vi "F Dwf Analog Impedance Reference Get.vi"(8 "error in (no error)":errorcluster, 10 "pohms":dbl, 11 "hdwf":i32) -> (0 "error out":errorcluster, 2 "pohms out":dbl, 3 "function return":i32)   [LabVIEW 2019, in "Olasdwf.lvlib"]
doc: "DWFAPI int FDwfAnalogImpedanceReferenceGet(HDWF hdwf, double *pohms);"
uses:
  Olasdwf.lvlib
  Windows/System32/dwf.dll
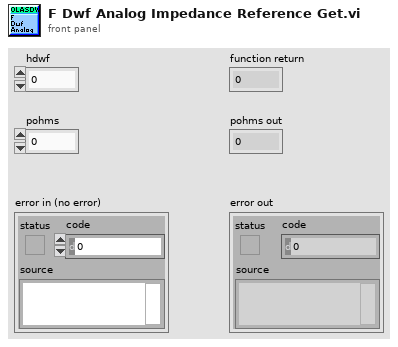
[diagram p1: front panel]
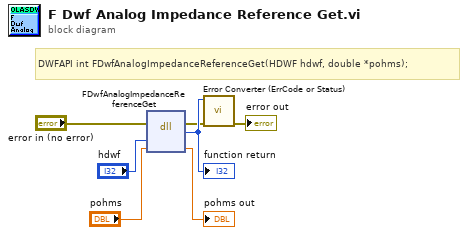
[diagram p0: block diagram]
diagram:
  # "DWFAPI int FDwfAnalogImpedanceReferenceGet(HDWF hdwf, double *pohms);"
  n1 = dll-call lib="C:/Windows/System32/dwf.*" fn="FDwfAnalogImpedanceReferenceGet"(error in="error in (no error)", "hdwf"="hdwf", "pohms"="pohms") -> (error out=w2:errorcluster, w7:i32, "pohms"=→"pohms out":dbl)  [unwired: 3 in, 1 out]
  "function return" <- w7
  n2 = call "Error Converter (ErrCode or Status).vi"("error in (no error)"=w2, "error code"=w7) -> ("error out"=→"error out":errorcluster)  [unwired: 9 in]
